vi "TripandIgnore.vi"(1 "Eval Period (s)":dbl, 2 "Signal In":bool) -> (0 "Tripped?":bool)   [LabVIEW 2016]
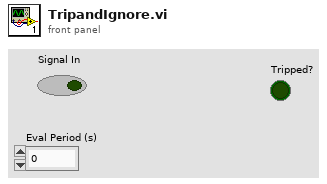
[diagram p1: front panel]
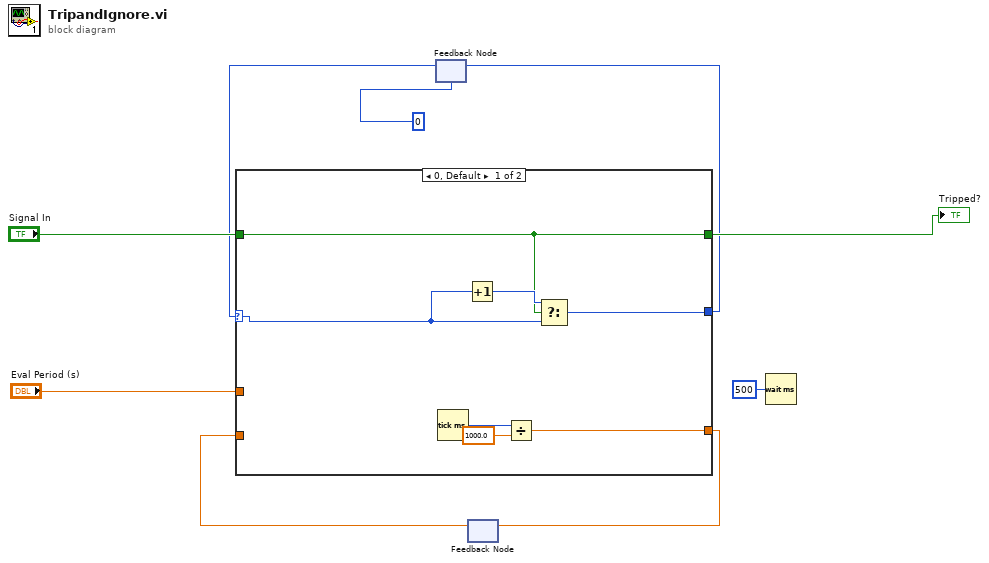
[diagram p0: block diagram]
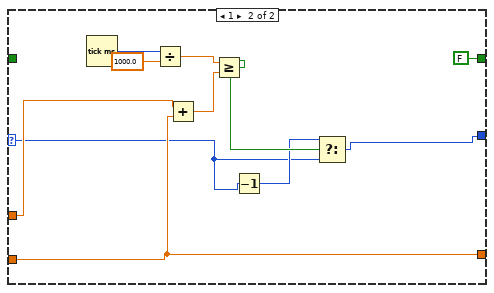
[diagram p2: hidden frame]
diagram:
  n1 = feedback #1(0) -> (w5:i32)
  n2 = feedback #2() -> (w2:dbl)  [unwired: 1 in]
  n3 = case shown="0, Default" w5 {
    selector: w5 -> [w16 w17]
    tunnel: "Signal In" -> [w10 _]
    tunnel: [w10 FALSE ("Output")] -> w8
    tunnel: [w14 w20] -> w7
    tunnel: "Eval Period (s)" -> [_ w23]
    tunnel: [w11 w22] -> w3
    tunnel: w2 -> [_ w22]
    frame 0, Default {
      n4 = Tick Count (ms)() -> (millisecond timer value=w13:u32)
      n5 = Increment(x=w16) -> (x+1=w15:i32)
      n6 = Divide(x=w13, y=1000.0) -> (x/y=w11:dbl)
      n7 = Select(t=w15, s=w10, f=w16) -> (s? t:f=w14:i32)
    }
    frame 1 {
      n8 = Tick Count (ms)() -> (millisecond timer value=w27:u32)
      n9 = Divide(x=w27, y=1000.0) -> (x/y=w25:dbl)
      n10 = Add(x=w23, y=w22) -> (x+y=w24:dbl)
      n11 = Greater Or Equal?(x=w25, y=w24) -> (x >= y?=w21:bool)
      n12 = Decrement(x=w17) -> (x-1=w18:i32)
      n13 = Select(t=w18, s=w21, f=w17) -> (s? t:f=w20:i32)
    }
  }
  "Tripped?" <- w8
  n14 = feedback-in #1(w7) -> ()
  n15 = feedback-in #2(w3) -> ()
  n16 = Wait (ms)(milliseconds to wait=u32 500) -> ()  [unwired: 1 out]
